vi "spectral_measurement.vi"(0 "Signals":waveform(sgl)[](array[waveform]), 2 "Restart Averaging":bool, 7 "error in (no error)":errorcluster, 12 "dB On":bool=TRUE, 13 "Spectrum Averaging Parameters":T2={"averaging mode"=2, "weighting mode"=1, "number of averages"=0} {"averaging mode" items=["No averaging", "Vector averaging", "RMS averaging", "Peak hold"]; "weighting mode" items=["Linear", "Exponential"]}, 14 "Window":T1(ring)=enum."Hanning") -> (8 "PSD":cluster{"f0":dbl, "df":dbl, "magnitude":dbl[]}[](array[cluster]), 9 "averaging done":bool, 11 "error out":errorcluster)   [LabVIEW 2014]
uses:
  <vilib>/express/express analysis/Spectral/Block/exnSpectralBlock spectral measurements PSD array WFM.vi
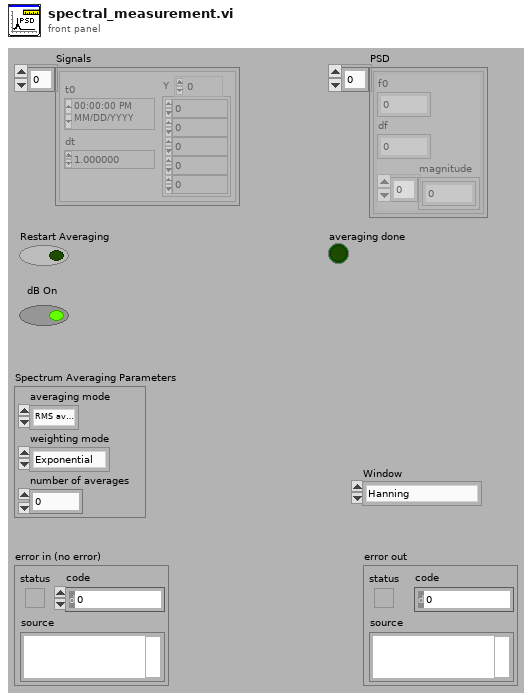
[diagram p1: front panel]
types:
  T1 = enum16{"None ", "Hanning", "Hamming", "Blackman-Harris", "Exact Blackman", "Blackman", "Flat Top", "4 Term B-Harris ", "7 Term B-Harris", "Low Sidelobe"}
  T2 = cluster{"averaging mode":u16, "weighting mode":u16, "number of averages":u32}
  T3 = cluster{"dB On (F)":bool, "unwrap phase (F)":bool, "convert to degree (F)":bool}
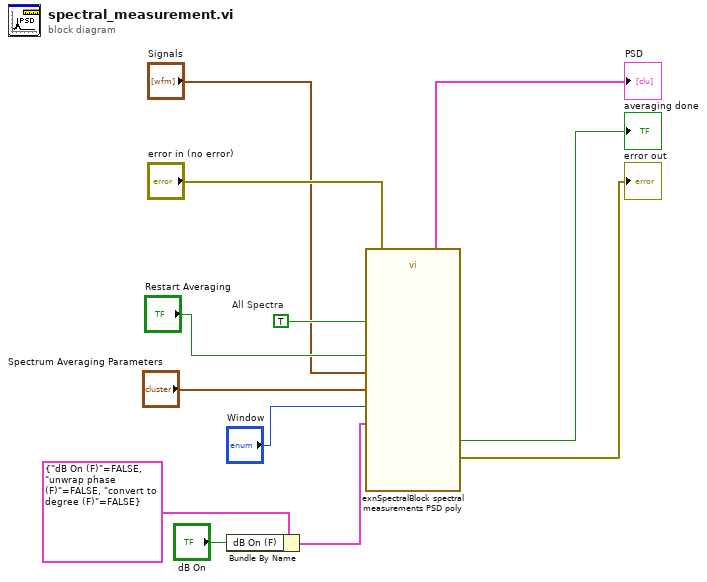
[diagram p0: block diagram]
diagram:
  w11 = TRUE  # All Spectra
  n1 = Bundle By Name(cluster=T3 {"dB On (F)"=FALSE, "unwrap phase (F)"=FALSE, "convert to degree (F)"=FALSE} ("View"), "dB On (F)"="dB On") -> (w2:T3)
  n2 = call-poly <vilib>:"exnSpectralBlock spectral measurements PSD poly.vi"("Signals"="Signals", "Restart Averaging"="Restart Averaging", "View"=w2, "Spectrum Window"="Window", "error in (no error)"="error in (no error)", "Spectrum Averaging Parameters"="Spectrum Averaging Parameters", "All Spectra"=w11) -> ("Measurement Output"=→"PSD":cluster{"f0":dbl, "df":dbl, "magnitude":dbl[]}[], "averaging done"=→"averaging done":bool, "error out"=→"error out":errorcluster)  [unwired: 6 in]
